vi "MicroPVHTML100_2.vi"(8 "errin":errorcluster caption="entrée d'erreur (pas d'erreur)", 11 "path in":path) -> (0 "sortie d'erreur":errorcluster, 1 "Numérique":i32, 2 "Tableau":string[][](array[string]), 3 "tableau":string[][](array[string]))   [LabVIEW 2020]
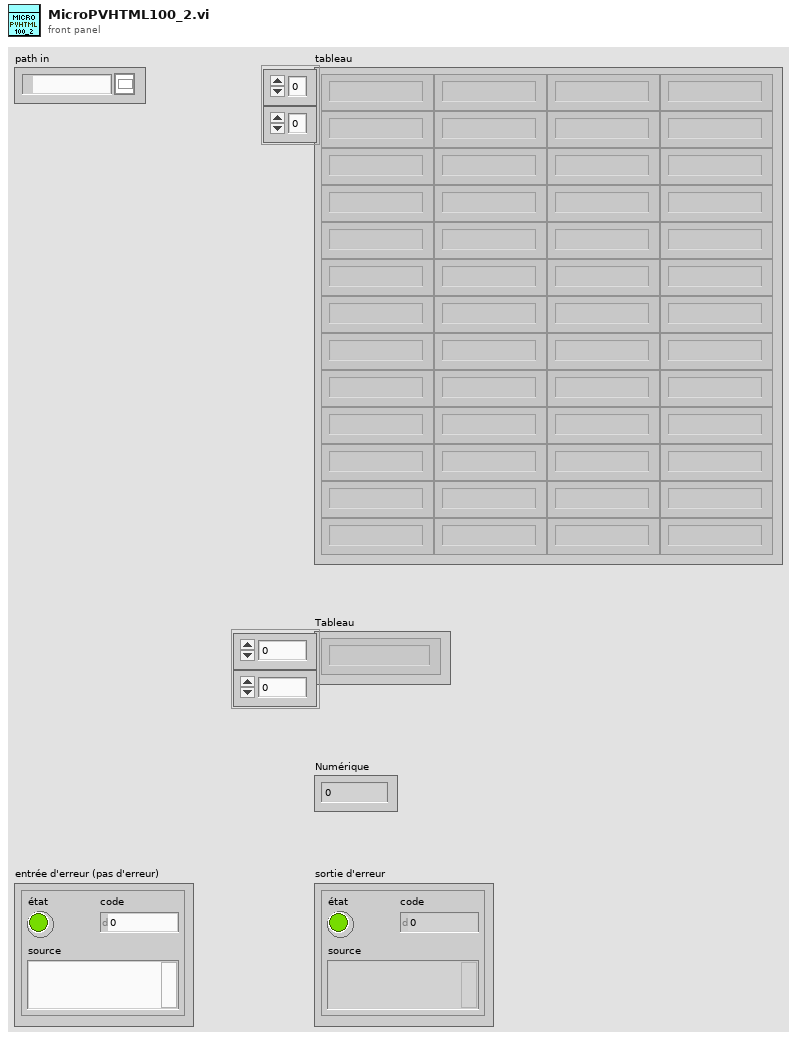
[diagram p1: front panel]
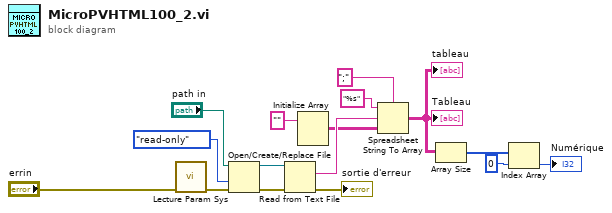
[diagram p0: block diagram]
diagram:
  n1 = call "Lecture Param Sys.vi"("errin"="errin") -> ("error out"=w15:errorcluster)  [unwired: 10 in]
  n2 = Open/Create/Replace File(file path (use dialog)="path in", error in=w15, access (0:read/write)=enum16{"read/write", "read-only", "write-only"}."read-only" ("accès (0 : read/write)")) -> (refnum out=w12:refnum<file>, error out=w2:errorcluster)  [unwired: 3 in, 1 out]
  n3 = Read from Text File(file (use dialog)=w12, error in=w2) -> (text=w6:string, error out=→"sortie d'erreur":errorcluster)  [unwired: 2 in, 2 out]
  n4 = Initialize Array("") -> (w4:string[][])  [unwired: 2 in]
  n5 = Spreadsheet String To Array(delimiter (Tab)=";" ("séparateur (Tabulation)"), format string="%s" ("chaîne de format"), spreadsheet string=w6, array type (2D Dbl)=w4) -> (array=w16:string[][])
  "tableau" <- w16
  "Tableau" <- w16
  n6 = Array Size(array=w16) -> (size(s)=w8:i32[])
  n7 = Index Array(array=w8, index=0 ("indice")) -> (element=→"Numérique":i32)
